vi "Lookup Queue Actor ID.vi"(8 "error in (no error)":errorcluster, 10 "Actor ID":string, 11 "Actor Monitor in":refnum<class "Actor Monitor.lvclass">) -> (0 "error out":errorcluster, 2 "Actor's Queue":refnum<class "Message Enqueuer.lvclass">, 3 "Actor Monitor out":refnum<class "Actor Monitor.lvclass">)   [LabVIEW 2018, in "Monitored Actor.lvlib" / "Actor Monitor.lvclass"]
doc: "Uses the actor ID to lookup the actor's queue\n\nCopyright: MGI\nAuthored by: Derek Trepanier"
uses:
  Actor Monitor.lvclass
  <vilib>/ActorFramework/Message Enqueuer/Message Enqueuer.lvclass
  Actor Monitor.lvclass/Actor Monitor.ctl
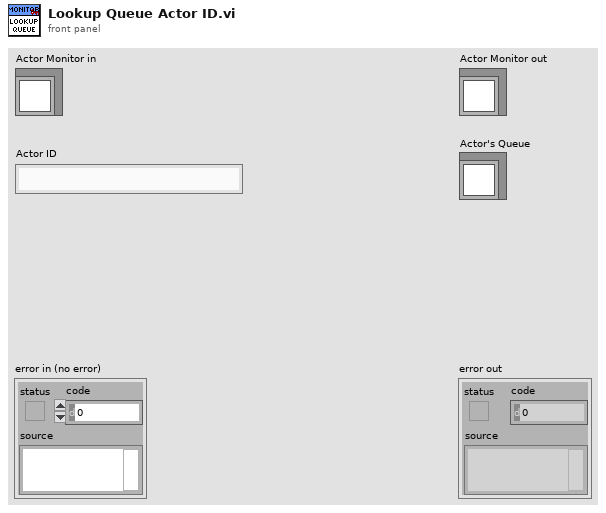
[diagram p1: front panel]
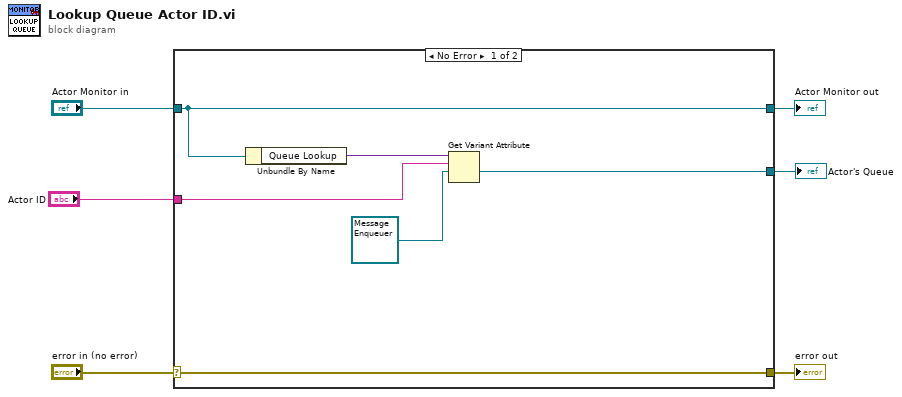
[diagram p0: block diagram]
diagram:
  n1 = case shown="No Error" "error in (no error)" {
    selector: "error in (no error)" -> [w12 w14]
    tunnel: [w12 w14] -> w5
    tunnel: [w11 w13] -> w3
    tunnel: "Actor Monitor in" -> [w11 w13]
    tunnel: "Actor ID" -> [w9 _]
    tunnel: [w7 _] -> w1
    frame No Error {
      n2 = Unbundle By Name(w11) -> ("Queue Lookup"=w10:variant)
      n3 = Get Variant Attribute(Variant=w10, name=w9, default value (empty Variant)=refnum<class "Message Enqueuer.lvclass"> refnum ("Caller Enqueuer")) -> (value=w7:refnum<class "Message Enqueuer.lvclass">)  [unwired: 1 in, 3 out]
    }
    frame Error {
    }
  }
  "error out" <- w5
  "Actor Monitor out" <- w3
  "Actor's Queue" <- w1
